vi "GenerateMenu.vi"(8 "error in":errorcluster, 10 "menu ref in":refnum<k9>, 11 "NISE_CEF_Repository in":refnum<class "NISE_CEF_Repository.lvclass">) -> (0 "error out":errorcluster, 2 "menu ref out":refnum<k9>, 3 "NISE_CEF_Repository out":refnum<class "NISE_CEF_Repository.lvclass">)   [LabVIEW 2013, in "NISE_CEF_Repository.lvclass"]
uses:
  NISE_CEF_Repository.lvclass
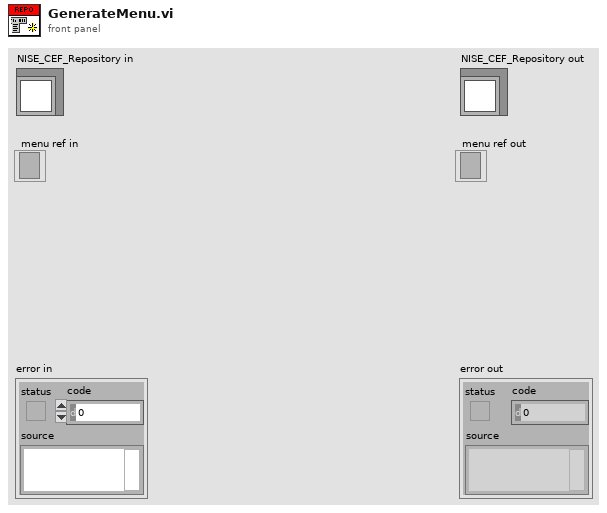
[diagram p1: front panel]
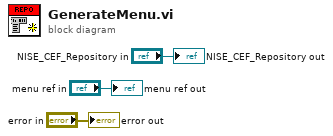
[diagram p0: block diagram]
diagram:
  "error out" <- "error in"
  "NISE_CEF_Repository out" <- "NISE_CEF_Repository in"
  "menu ref out" <- "menu ref in"
